vi "BaseTemplate_4x4x4_GetClassAttributesToModify.vi"(8 "error in (no error)":errorcluster, 9 "timeout (15000 ms)":i32=15000, 11 "reference in":refnum<class "BaseTemplate_4x4x4.lvclass">) -> (0 "error out":errorcluster, 1 "Timeout":bool, 2 "Class attributes":T1, 3 "reference out":refnum<class "BaseTemplate_4x4x4.lvclass">)   [LabVIEW 2020, in "BaseTemplate_4x4x4.lvclass"]
doc: "This VI returns the class attributes associated with the object reference and places a lock on the object. If reference is wired, the class attributes of this class (or sub class) will be returned else the class attributes will default to the class.\n\nIf the object is currently locked for modification by another method, 'Timeout' specifies how long the VI should wait to receive access to the object. The default value waits until the object becomes available.\n\nYou must use this class SetModifiedClassAttributes VI to set the object's data and release the lock."
uses:
  <resource>/Framework/Providers/Open_GDS/ClassProviders/Provider_EndevoGOOP300/Templates/BaseTemplate_4x4x4/BaseTemplate_4x4x4.lvclass
  <resource>/Framework/Providers/Open_GDS/ClassProviders/Provider_EndevoGOOP300/Templates/BaseTemplate_4x4x4/protected/ClassAttributes.ctl
  <vilib>/addons/_goop3.llb/3GOOPStates.ctl
  <resource>/Framework/Providers/Open_GDS/ClassProviders/Provider_EndevoGOOP300/Templates/BaseTemplate_4x4x4/BaseTemplate_4x4x4.lvclass/BaseTemplate_4x4x4.ctl
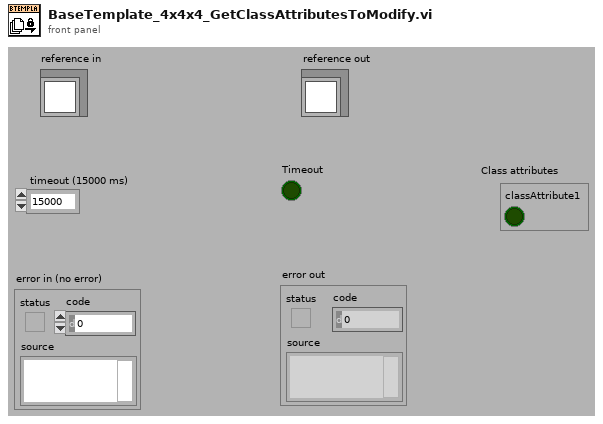
[diagram p1: front panel]
types:
  T1 = typedef "BaseTemplate_4x4x4.lvclass/ClassAttributes.ctl" = cluster{"classAttribute1":bool}
  T2 = typedef "3GOOPStates.ctl" = enum16{"Set", "Get", "New", "Delete", "Clear", "Test and get", "Unlock data", "Information", "Look up existing", "New or look up existing", "Test and get shared", "Get shared", "Set shared", "Unlock shared", "Find dynamic method", "Register dynamic method", "Preload dynamic method", "Probe", "Cast to more generic", "Cast to more specific"}
  T3 = typedef "BaseTemplate_4x4x4.lvclass/ObjectReference.ctl" = refnum<k1>
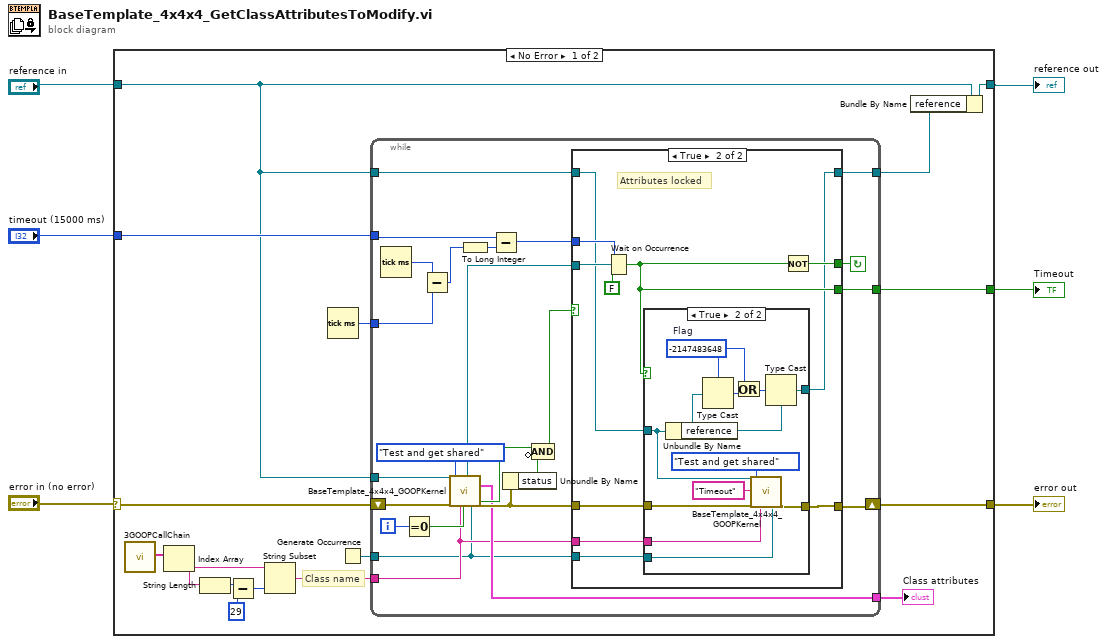
[diagram p0: block diagram]
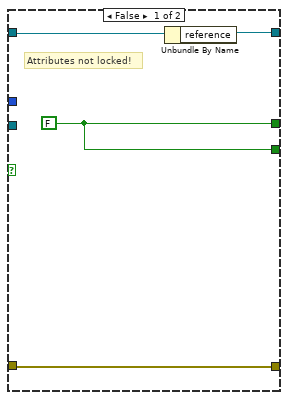
[diagram p2: hidden frame]
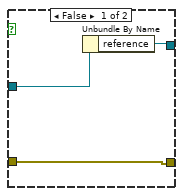
[diagram p3: hidden frame]
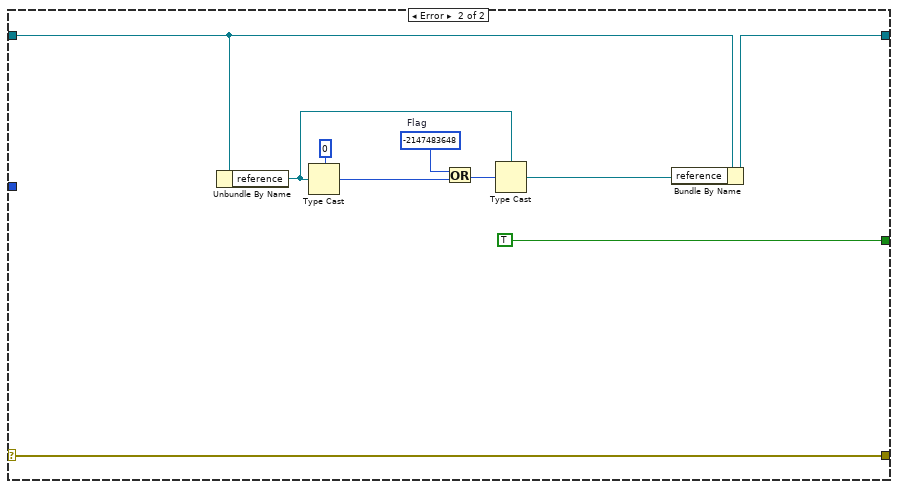
[diagram p4: hidden frame]
diagram:
  n1 = case shown="No Error" "error in (no error)" {
    selector: "error in (no error)" -> [w19 w86]
    tunnel: [w16 w82] -> w3
    tunnel: [w18 w86] -> w6
    tunnel: "reference in" -> [w15 w83]
    tunnel: [w17 TRUE ("timed out")] -> w5
    tunnel: "timeout (15000 ms)" -> [w20 _]
    frame No Error {
      # "Class name"
      n2 = call <vilib>:"3GOOPCallChain.vi"() -> ("call chain"=w8:string[])
      n3 = Index Array(array=w8) -> (element=w9:string)  [unwired: 1 in]
      n4 = String Length(string=w9) -> (length=w12:i32)
      n5 = Subtract(x=w12, y=29) -> (x-y=w10:i32)
      n6 = String Subset(string=w9, length (rest)=w10) -> (substring=w7:string)  [unwired: 1 in]
      n7 = Tick Count (ms)() -> (millisecond timer value=w21:u32)
      n8 = Generate Occurrence() -> (w22:refnum<k4>)
      n9 = while {
        tunnel: [w25] -> w13
        shift-left: w19 -> [w43]
        shift-right: [w29] -> w18
        tunnel: [w45] -> w17
        tunnel: w20 -> [w35]
        tunnel: w15 -> [w44]
        tunnel: w22 -> [w23]
        tunnel: w21 -> [w26]
        tunnel: w15 -> [w31]
        tunnel: [w28] -> w14
        tunnel: w7 -> [w24]
        i -> [w39]
        stop <- w46 continue-if-true
        n10 = Tick Count (ms)() -> (millisecond timer value=w27:u32)
        n11 = Equal To 0?(x=w39) -> (x = 0?=w38:bool)
        n12 = Subtract(x=w27, y=w26) -> (x-y=w34:u32)
        n13 = call <resource>:"BaseTemplate_4x4x4_GOOPKernel.vi"("Ref in"=w44, "error in (no error)"=w43, "Action"=3GOOPStates."Test and get shared", "Class name"=w24, "Misc"=w38, "Occurrence shared"=w23) -> ("Occurrence out"=w37:refnum<k4>, "Data shared out"=w25:T1, "Data locked?"=w41:bool, "error out"=w30:errorcluster)  [unwired: 11 in, 7 out]
        n14 = To Long Integer(number=w34) -> (32bit integer=w32:i32)
        n15 = Subtract(x=w35, y=w32) -> (x-y=w33:i32)
        n16 = Unbundle By Name(w30) -> ("status"=w42:bool)
        n17 = Compound Arithmetic op=AND(w41, invert w42) -> (w40:bool)
        n18 = case shown="True" w40 {
          tunnel: w37 -> [_ w60]
          tunnel: w33 -> [_ w58]
          tunnel: [w50 w61] -> w46
          tunnel: [w50 w54] -> w45
          tunnel: w31 -> [w48 w57]
          tunnel: w30 -> [w49 w56]
          tunnel: [w49 w55] -> w29
          tunnel: w23 -> [_ w53]
          tunnel: [w47 w52] -> w28
          tunnel: w24 -> [_ w51]
          frame False {
            w50 = FALSE
            # "Attributes not locked!"
            n19 = Unbundle By Name(w48) -> ("reference"=w47:T3)
          }
          frame True {
            # "Attributes locked"
            n20 = Wait on Occurrence(1:FALSE ("ignore previous (T)"), 2:w60, 3:w58) -> (0:w54:bool)
            n21 = case shown="True" w54 {
              tunnel: w57 -> [w63 w71]
              tunnel: w56 -> [w64 w76]
              tunnel: [w64 w75] -> w55
              tunnel: w53 -> [_ w65]
              tunnel: [w62 w69] -> w52
              tunnel: w51 -> [_ w66]
              frame False {
                n22 = Unbundle By Name(w63) -> ("reference"=w62:T3)
              }
              frame True {
                w67 = -2147483648  # Flag
                n23 = Unbundle By Name(w71) -> ("reference"=w70:T3)
                n24 = Type Cast(type=w67, x=w70) -> (*(type *) &x=w72:i32)
                n25 = Or(x=w67, y=w72) -> (x .or. y?=w68:i32)
                n26 = call <resource>:"BaseTemplate_4x4x4_GOOPKernel.vi"("Ref in"=w71, "Probe in"="Timeout" ("VI ref"), "error in (no error)"=w76, "Action"=3GOOPStates."Test and get shared", "Class name"=w66, "Occurrence shared"=w65) -> ("error out"=w75:errorcluster)  [unwired: 11 in, 10 out]
                n27 = Type Cast(type=w70, x=w68) -> (*(type *) &x=w69:T3)
              }
            }
            n28 = Not(x=w54) -> (.not. x?=w61:bool)
          }
        }
      }
      "Class attributes" <- w13
      n29 = Bundle By Name(cluster=w15, "reference"=w14) -> (w16:refnum<class "BaseTemplate_4x4x4.lvclass">)
    }
    frame Error {
      w84 = -2147483648  # Flag
      n30 = Unbundle By Name(w83) -> ("reference"=w77:T3)
      n31 = Type Cast(type=0, x=w77) -> (*(type *) &x=w80:i32)
      n32 = Or(x=w84, y=w80) -> (x .or. y?=w79:i32)
      n33 = Type Cast(type=w77, x=w79) -> (*(type *) &x=w78:T3)
      n34 = Bundle By Name(cluster=w83, "reference"=w78) -> (w82:refnum<class "BaseTemplate_4x4x4.lvclass">)
    }
  }
  "error out" <- w6
  "reference out" <- w3
  "Timeout" <- w5
